vi "Setup Example SCD.vi"(8 "error in (no error)":errorcluster, 11 "SCD in":refnum<class "SCD.lvclass">) -> (0 "error out":errorcluster, 1 "device is open?":bool, 2 "Module Was Already Running?":bool, 3 "SCD out":refnum<class "SCD.lvclass">)   [LabVIEW 2023, in "Examples.lvlib"]
doc: "Setup for the mono examples."
uses:
  Examples.lvlib
  Classes/DeviceManager/DeviceManager.lvlib
  Classes/SCD/SCD.lvclass
panel:
  # "Connector Pane"
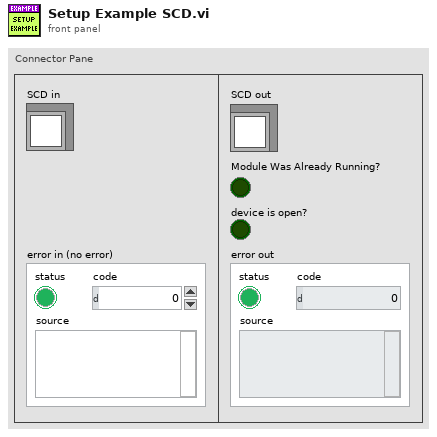
[diagram p1: front panel]
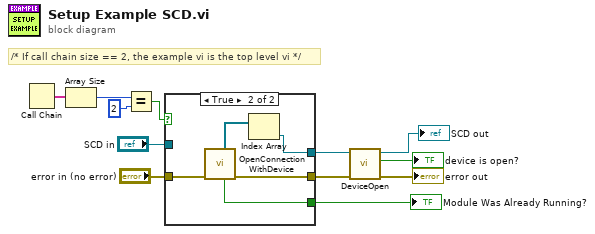
[diagram p0: block diagram]
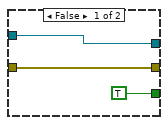
[diagram p2: hidden frame]
diagram:
  # "/* If call chain size == 2, the example vi is the top level vi */"
  n1 = Call Chain() -> (call chain=w9:string[])
  n2 = Array Size(array=w9) -> (size(s)=w10:i32)
  n3 = Equal?(x=w10, y=2) -> (x = y?=w12:bool)
  n4 = case shown="True" w12 {
    tunnel: [w15 w19] -> w6
    tunnel: "SCD in" -> [w15 _]
    tunnel: [TRUE ("Module Was Already Running?") w20] -> w8
    tunnel: "error in (no error)" -> [w14 w18]
    tunnel: [w14 w17] -> w5
    frame False {
    }
    frame True {
      n5 = call "OpenConnectionWithDevice.vi"("error in"=w18) -> ("error out"=w17:errorcluster, "Module Was Already Running?"=w20:bool, "SCDs"=w16:refnum<class "SCD.lvclass">[])  [unwired: 6 in, 2 out]
      n6 = Index Array(array=w16) -> (element=w19:refnum<class "SCD.lvclass">)  [unwired: 1 in]
    }
  }
  "Module Was Already Running?" <- w8
  n7 = call-dynamic "DeviceOpen.vi"("error in (no error)"=w5, "SCD in"=w6) -> ("error out"=→"error out":errorcluster, "device is open?"=→"device is open?":bool, "SCD out"=→"SCD out":refnum<class "SCD.lvclass">)  [unwired: 6 in, 1 out]
